vi "Get Event Structure Num.vi"(8 "error in (no error)":errorcluster, 11 "CSM-Helper in":refnum<class "CSM-Helper.lvclass">) -> (0 "error out":errorcluster, 2 "EvtStruNum":i32, 3 "CSM-Helper out":refnum<class "CSM-Helper.lvclass">)   [LabVIEW 2020, in "CSM-Helper.lvclass"]
uses:
  CSM-Helper.lvclass
  CSM-Helper.lvclass/CSM-Helper.ctl
  Properties/Read Case Structure Ref.vi
  23d72305-f0a8-4ea4-80e2-b48919ab28b1.vi
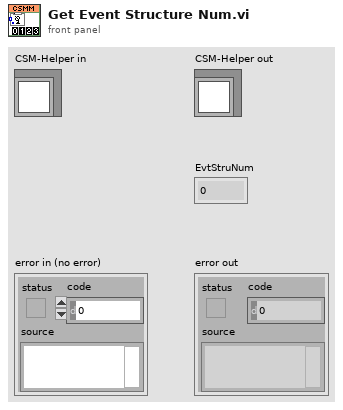
[diagram p1: front panel]
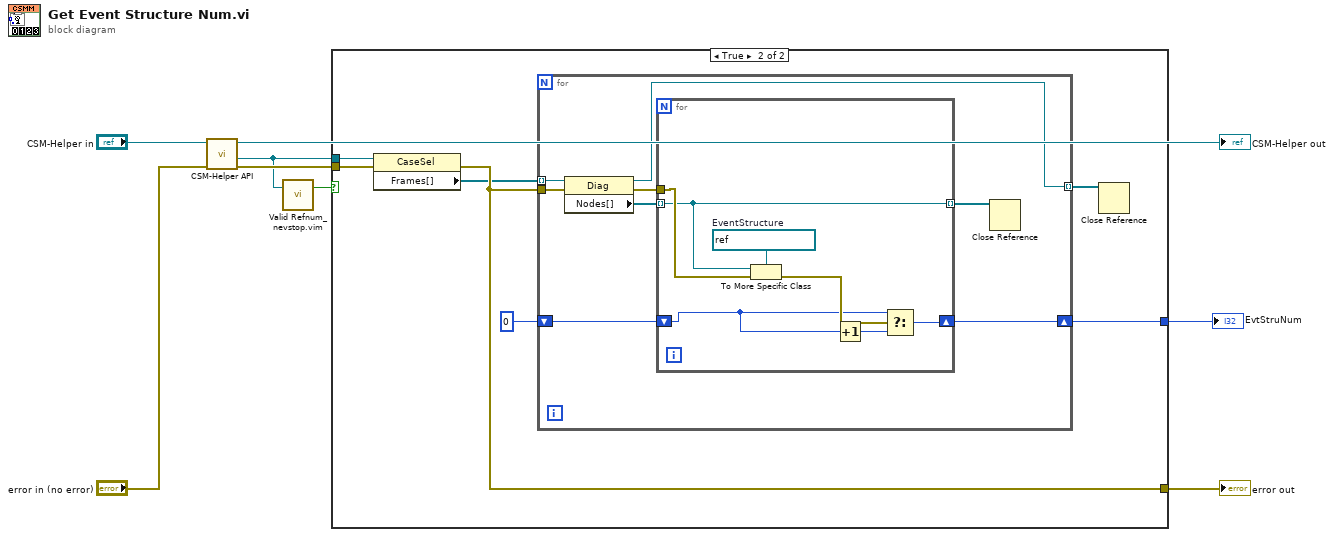
[diagram p0: block diagram]
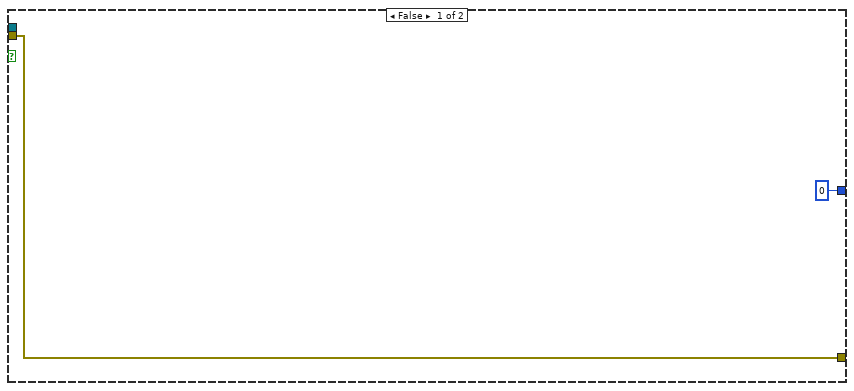
[diagram p2: hidden frame]
diagram:
  n1 = call-poly "CSM-Helper API.vi"("error in (no error)"="error in (no error)", "CSM-Helper in"="CSM-Helper in") -> ("error out"=w5:errorcluster, "Case Structure"=w2:refnum<vi>, "CSM-Helper out"=→"CSM-Helper out":refnum<class "CSM-Helper.lvclass">)  [unwired: 7 in]
  n2 = call "Valid Refnum_nevstop.vim"("number/path/refnum"=w2) -> ("Valid Number/Path/Refnum"=w1:bool)  [unwired: 2 in]
  n3 = case shown="True" w1 {
    tunnel: w5 -> [w10 w17]
    tunnel: [0 w15] -> w4
    tunnel: [w10 w14] -> w3
    tunnel: w2 -> [_ w11]
    frame False {
    }
    frame True {
      n4 = property class="CaseSel"(reference=w11, error in=w17) -> (error out=w14:errorcluster, "Frames[]"=w13:refnum<vi>[])  [unwired: 1 out]
      n5 = for {
        tunnel: w13 -> [w25] mode=indexing
        shift-right: [w23] -> w15
        shift-left: 0 -> [w24]
        tunnel: w14 -> [w21]
        tunnel: [w18] -> w12 mode=indexing
        n6 = property class="Diag"(reference=w25, error in=w21) -> (reference out=w18:refnum<vi>, error out=w20:errorcluster, "Nodes[]"=w22:refnum<vi>[])
        n7 = for {
          tunnel: w22 -> [w26] mode=indexing
          shift-right: [w31] -> w23
          shift-left: w24 -> [w29]
          tunnel: w20 -> [w27]
          tunnel: [w26] -> w19 mode=indexing
          w32 = refnum<vi> refnum  # EventStructure
          n8 = To More Specific Class(target class=w32, reference=w26, error in=w27) -> (error out=w30:errorcluster)  [unwired: 1 out]
          n9 = Increment(x=w29) -> (x+1=w28:i32)
          n10 = Select(t=w29, s=w30, f=w28) -> (s? t:f=w31:i32)
        }
        n11 = Close Reference(reference=w19) -> ()  [unwired: 1 in, 1 out]
      }
      n12 = Close Reference(reference=w12) -> ()  [unwired: 1 in, 1 out]
    }
  }
  "error out" <- w3
  "EvtStruNum" <- w4
